vi "Autonomous.vi"   [LabVIEW 2016]
doc: "This VI starts when autonomous period begins, and will automatically be terminated when it ends. You can carry out timed or sensor driven operations directly to I/O or to subsystems without needing to return to the caller."
uses:
  <vilib>/Rock Robotics/WPI/Utilities/WPI_GetSetVariantRefNum.vi
  <vilib>/Rock Robotics/Network Tables/NT Read String.vi
types:
  T1 = typedef "WPI_DriverStationPositionInfo.ctl" = enum16{"1", "2", "3"}
  T2 = typedef "WPI_JoystickDevRef.ctl" = cluster{"Device":T3}
  T3 = typedef "WPI_JoystickDeviceEnum.ctl" = enum16{"USB 0", "USB 1", "USB 2", "USB 3", "USB 4", "USB 5"}
  T4 = typedef "Command Status Info.ctl" = cluster{"Name":string, "Status":T5, "notifier out":T6}
  T5 = typedef "Completion Status.ctl" = enum16{"Successful", "Aborted", "Incomplete"}
  T6 = typedef "Completion Notifier.ctl" = refnum<notifier>
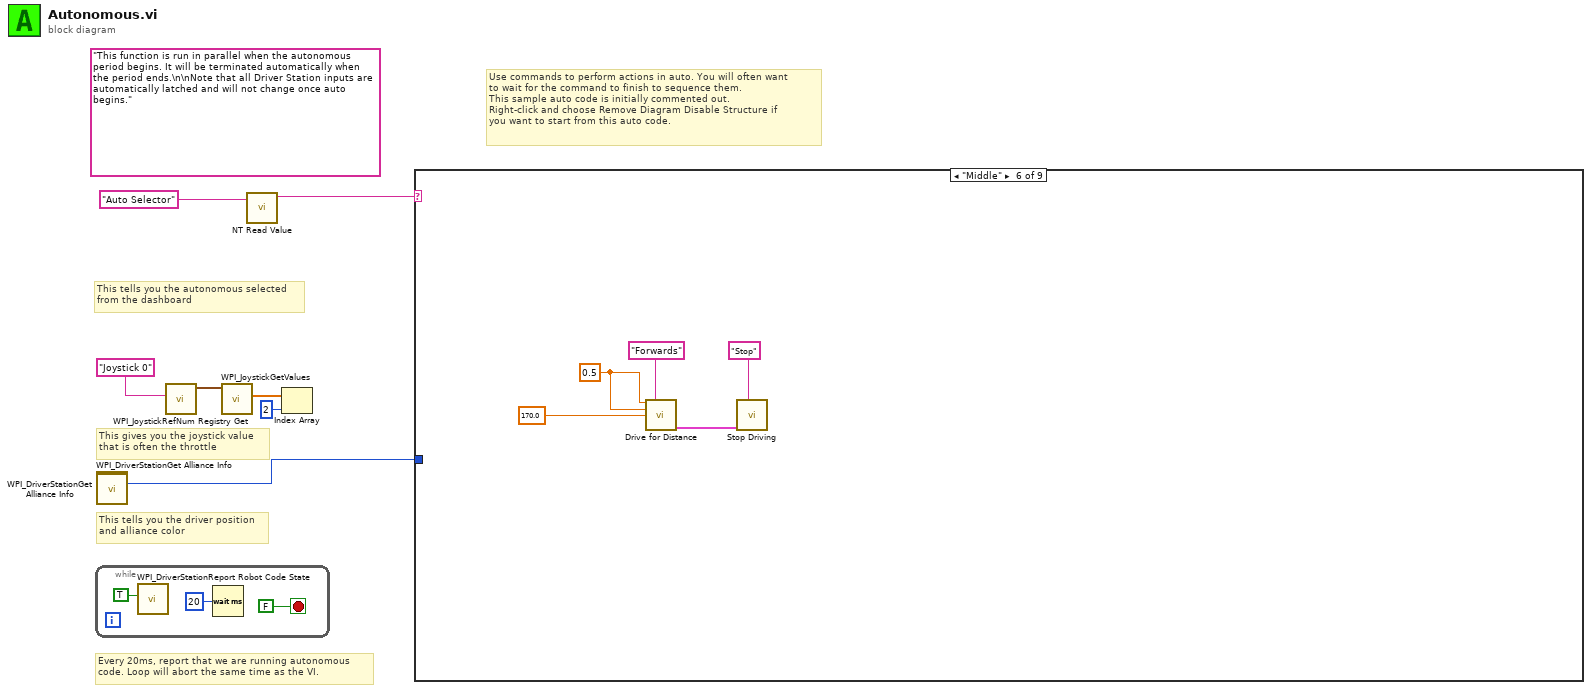
[diagram p0: block diagram]
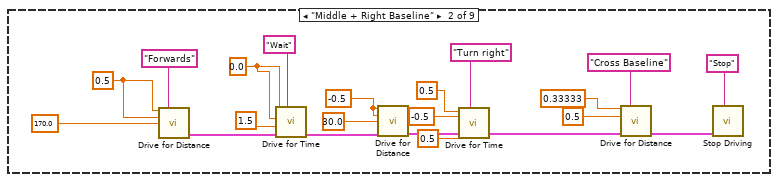
[diagram p3: hidden frame]
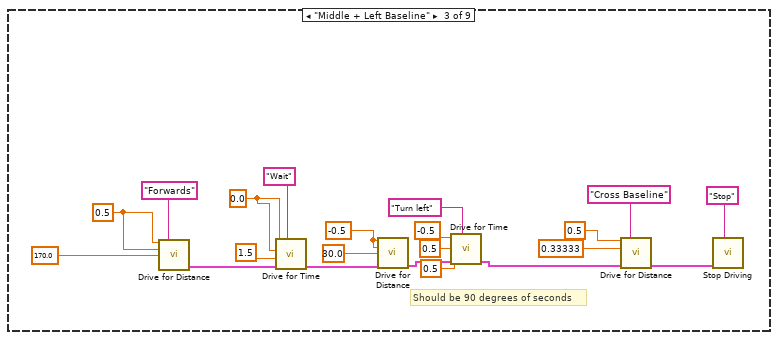
[diagram p4: hidden frame]
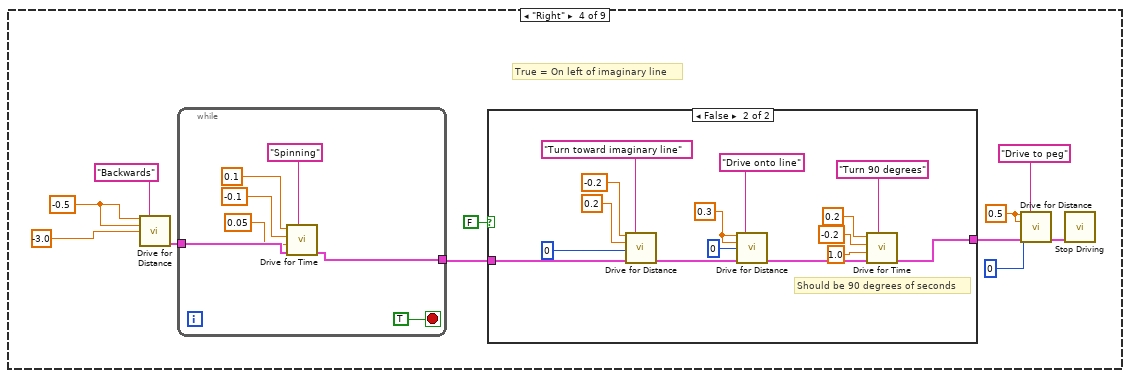
[diagram p5: hidden frame]
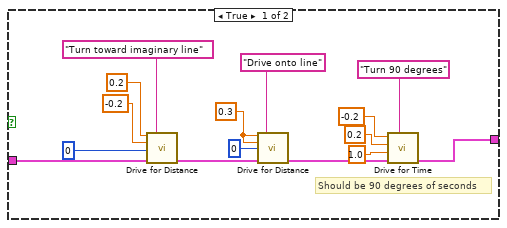
[diagram p6: hidden frame]
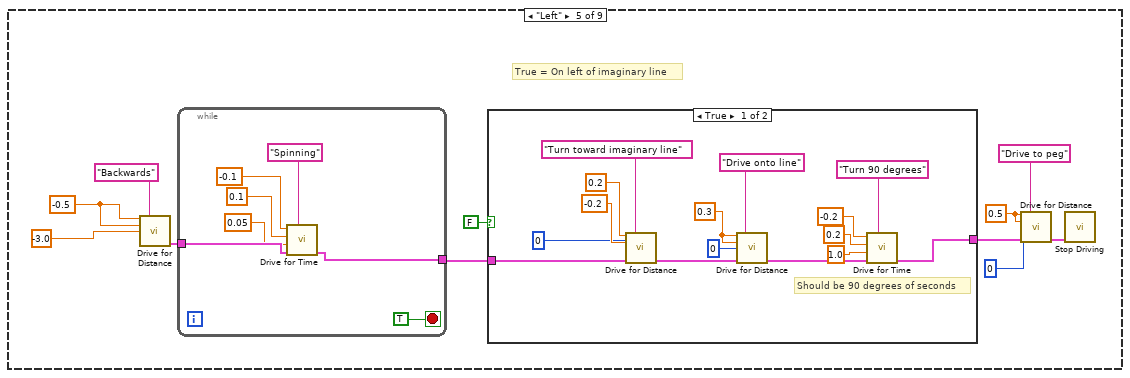
[diagram p7: hidden frame]
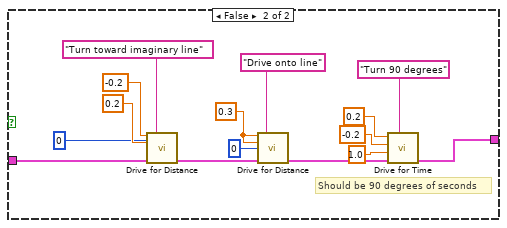
[diagram p8: hidden frame]
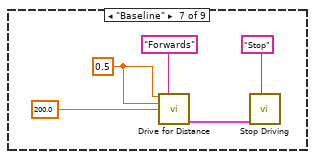
[diagram p9: hidden frame]
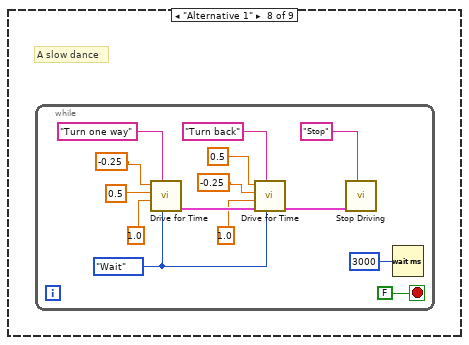
[diagram p10: hidden frame]
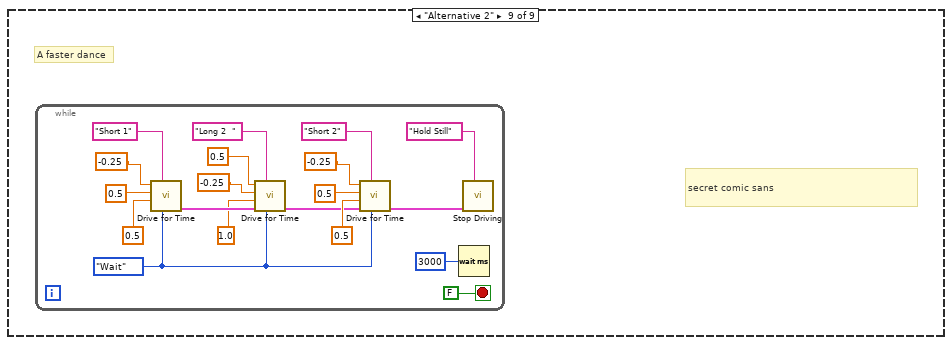
[diagram p11: hidden frame]
diagram:
  (unwired) "This function is run in parallel when the autonomous period begins. It will be terminated automatically when the period ends.\n\nNote that all Driver Station inputs are automatically latched and will not change once auto begins."
  # "This tells you the autonomous selected\nfrom the dashboard"
  # "Every 20ms, report that we are running autonomous\ncode. Loop will abort the same time as the VI."
  # "This gives you the joystick value\nthat is often the throttle"
  # "Use commands to perform actions in auto. You will often want\nto wait for the command to finish to sequence them.\nThis sample auto code is initially commented out. \nRight-click and choose Remove Diagram Disable Structure if\nyou want to start from this auto code."
  # "This tells you the driver position\nand alliance color"
  n1 = while {
    stop <- FALSE stop-if-true
    n2 = call <vilib>:"WPI_DriverStationReport Robot Code State.vi"("Autonomous"=TRUE) -> ()  [unwired: 10 in, 1 out]
    n3 = Wait (ms)(milliseconds to wait=u32 20) -> ()  [unwired: 1 out]
  }
  n4 = call <vilib>:"WPI_DriverStationGet Alliance Info.vi"() -> ("Position"=w1:T1)  [unwired: 11 out]
  n5 = call <vilib>:"WPI_DriverStationGet Alliance Info.vi"() -> ()  [unwired: 12 out]
  n6 = call <vilib>:"WPI_JoystickRefNum Registry Get.vi"("refnum name"="Joystick 0") -> ("JoystickDevRef"=w6:T2)  [unwired: 1 in, 9 out]
  n7 = call <vilib>:"WPI_JoystickGetValues.vi"("JoystickDevRef"=w6) -> ("Axes"=w5:dbl[])  [unwired: 6 in, 4 out]
  n8 = call-poly <vilib>:"NT Read Value.vi"("Name"="Auto Selector") -> ("String"=w2:string)  [unwired: 9 in, 1 out]
  n9 = Index Array(array=w5, index=2) -> ()  [unwired: 1 out]
  n10 = case shown="\"Middle\"" w2 {
    tunnel: w1 -> [_ _ _ _ _ _ _ _ _]
    frame Default {
      # "You can put your main auto here, or you can right-click on the case and make any\nother frame be the default case."
      # "This is the frame that will execute if no selection is made, or if it is not recognized"
    }
    frame "Middle + Right Baseline" {
      w22 = -0.5 ("Left Setpoint")
      w25 = 0.0 ("Left Speed")
      w30 = 0.5
      n11 = call "Drive for Distance.vi"("Left Setpoint"=w30, "Description"="Forwards", "Right Setpoint"=w30, "Distance"=170.0) -> ("Command Info Out"=w27:T4)  [unwired: 11 in]
      n12 = call "Drive for Time.vi"("Description"="Wait", "Command Info In"=w27, "Seconds"=1.5, "Right Speed"=w25, "Left Speed"=w25) -> ("Command Info Out"=w21:T4)  [unwired: 5 in, 1 out]
      n13 = call "Drive for Distance.vi"("Left Setpoint"=w22, "Right Setpoint"=w22, "Distance"=30.0, "Command Info In"=w21) -> ("Command Info Out"=w16:T4)  [unwired: 11 in]
      n14 = call "Drive for Time.vi"("Description"="Turn right", "Command Info In"=w16, "Seconds"=0.5, "Right Speed"=-0.5 ("Angle"), "Left Speed"=0.5 ("Setpoint")) -> ("Command Info Out"=w12:T4)  [unwired: 5 in, 1 out]
      n15 = call "Drive for Distance.vi"("Left Setpoint"=0.33333, "Description"="Cross Baseline", "Right Setpoint"=0.5, "Command Info In"=w12) -> ("Command Info Out"=w17:T4)  [unwired: 11 in]
      n16 = call "Stop Driving.vi"("Description"="Stop", "Command Info In"=w17) -> ()  [unwired: 9 in, 1 out]
    }
    frame "Middle + Left Baseline" {
      w43 = -0.5 ("Left Setpoint")
      w46 = 0.0 ("Left Speed")
      w51 = 0.5
      # "Should be 90 degrees of seconds"
      n17 = call "Drive for Distance.vi"("Left Setpoint"=w51, "Description"="Forwards", "Right Setpoint"=w51, "Distance"=170.0) -> ("Command Info Out"=w48:T4)  [unwired: 11 in]
      n18 = call "Drive for Time.vi"("Description"="Wait", "Command Info In"=w48, "Seconds"=1.5, "Right Speed"=w46, "Left Speed"=w46) -> ("Command Info Out"=w42:T4)  [unwired: 5 in, 1 out]
      n19 = call "Drive for Distance.vi"("Left Setpoint"=w43, "Right Setpoint"=w43, "Distance"=30.0, "Command Info In"=w42) -> ("Command Info Out"=w37:T4)  [unwired: 11 in]
      n20 = call "Drive for Time.vi"("Description"="Turn left", "Command Info In"=w37, "Seconds"=0.5, "Right Speed"=0.5 ("Angle"), "Left Speed"=-0.5 ("Setpoint")) -> ("Command Info Out"=w36:T4)  [unwired: 5 in, 1 out]
      n21 = call "Drive for Distance.vi"("Left Setpoint"=0.5, "Description"="Cross Baseline", "Right Setpoint"=0.33333, "Command Info In"=w36) -> ("Command Info Out"=w38:T4)  [unwired: 11 in]
      n22 = call "Stop Driving.vi"("Description"="Stop", "Command Info In"=w38) -> ()  [unwired: 9 in, 1 out]
    }
    frame "Right" {
      w56 = 0.5 ("Left Setpoint")
      w62 = -0.5 ("Left Setpoint")
      # "True = On left of imaginary line"
      n23 = call "Drive for Distance.vi"("Left Setpoint"=w62, "Description"="Backwards", "Right Setpoint"=w62, "Distance"=-3.0) -> ("Command Info Out"=w60:T4)  [unwired: 11 in]
      n24 = while {
        tunnel: w60 -> [w100]
        tunnel: [w95] -> w59
        stop <- TRUE stop-if-true
        n25 = call "Drive for Time.vi"("Description"="Spinning", "Command Info In"=w100, "Seconds"=0.05, "Right Speed"=-0.1 ("Right Setpoint"), "Left Speed"=0.1 ("Left Setpoint")) -> ("Command Info Out"=w95:T4)  [unwired: 5 in, 1 out]
      }
      n26 = case shown="False" FALSE {
        tunnel: w59 -> [w78 w93]
        tunnel: [w64 w79] -> w57
        frame True {
          w70 = 0.3 ("Left Setpoint")
          # "Should be 90 degrees of seconds"
          n27 = call "Drive for Distance.vi"("Left Setpoint"=0.2, "Description"="Turn toward imaginary line", "Right Setpoint"=-0.2, "Distance"=0 ("temp (from vision)"), "Command Info In"=w78) -> ("Command Info Out"=w66:T4)  [unwired: 10 in]
          n28 = call "Drive for Distance.vi"("Left Setpoint"=w70, "Description"="Drive onto line", "Right Setpoint"=w70, "Distance"=0, "Command Info In"=w66) -> ("Command Info Out"=w72:T4)  [unwired: 10 in]
          n29 = call "Drive for Time.vi"("Description"="Turn 90 degrees", "Command Info In"=w72, "Seconds"=1.0, "Right Speed"=0.2 ("Right Setpoint"), "Left Speed"=-0.2 ("Left Setpoint")) -> ("Command Info Out"=w64:T4)  [unwired: 5 in, 1 out]
        }
        frame False {
          w85 = 0.3 ("Left Setpoint")
          # "Should be 90 degrees of seconds"
          n30 = call "Drive for Distance.vi"("Left Setpoint"=-0.2, "Description"="Turn toward imaginary line", "Right Setpoint"=0.2, "Distance"=0 ("temp (from vision)"), "Command Info In"=w93) -> ("Command Info Out"=w81:T4)  [unwired: 10 in]
          n31 = call "Drive for Distance.vi"("Left Setpoint"=w85, "Description"="Drive onto line", "Right Setpoint"=w85, "Distance"=0, "Command Info In"=w81) -> ("Command Info Out"=w87:T4)  [unwired: 10 in]
          n32 = call "Drive for Time.vi"("Description"="Turn 90 degrees", "Command Info In"=w87, "Seconds"=1.0, "Right Speed"=-0.2 ("Right Setpoint"), "Left Speed"=0.2 ("Left Setpoint")) -> ("Command Info Out"=w79:T4)  [unwired: 5 in, 1 out]
        }
      }
      n33 = call "Drive for Distance.vi"("Left Setpoint"=w56, "Description"="Drive to peg", "Right Setpoint"=w56, "Distance"=0, "Command Info In"=w57) -> ("Command Info Out"=w54:T4)  [unwired: 10 in]
      n34 = call "Stop Driving.vi"("Command Info In"=w54) -> ()  [unwired: 10 in, 1 out]
    }
    frame "Left" {
      w104 = 0.5 ("Left Setpoint")
      w110 = -0.5 ("Left Setpoint")
      # "True = On left of imaginary line"
      n35 = call "Drive for Distance.vi"("Left Setpoint"=w110, "Description"="Backwards", "Right Setpoint"=w110, "Distance"=-3.0) -> ("Command Info Out"=w108:T4)  [unwired: 11 in]
      n36 = while {
        tunnel: w108 -> [w148]
        tunnel: [w143] -> w107
        stop <- TRUE stop-if-true
        n37 = call "Drive for Time.vi"("Description"="Spinning", "Command Info In"=w148, "Seconds"=0.05, "Right Speed"=0.1 ("Right Setpoint"), "Left Speed"=-0.1 ("Left Setpoint")) -> ("Command Info Out"=w143:T4)  [unwired: 5 in, 1 out]
      }
      n38 = case shown="True" FALSE {
        tunnel: w107 -> [w126 w141]
        tunnel: [w112 w127] -> w105
        frame True {
          w118 = 0.3 ("Left Setpoint")
          # "Should be 90 degrees of seconds"
          n39 = call "Drive for Distance.vi"("Left Setpoint"=0.2, "Description"="Turn toward imaginary line", "Right Setpoint"=-0.2, "Distance"=0 ("temp (from vision)"), "Command Info In"=w126) -> ("Command Info Out"=w114:T4)  [unwired: 10 in]
          n40 = call "Drive for Distance.vi"("Left Setpoint"=w118, "Description"="Drive onto line", "Right Setpoint"=w118, "Distance"=0, "Command Info In"=w114) -> ("Command Info Out"=w120:T4)  [unwired: 10 in]
          n41 = call "Drive for Time.vi"("Description"="Turn 90 degrees", "Command Info In"=w120, "Seconds"=1.0, "Right Speed"=0.2 ("Right Setpoint"), "Left Speed"=-0.2 ("Left Setpoint")) -> ("Command Info Out"=w112:T4)  [unwired: 5 in, 1 out]
        }
        frame False {
          w133 = 0.3 ("Left Setpoint")
          # "Should be 90 degrees of seconds"
          n42 = call "Drive for Distance.vi"("Left Setpoint"=-0.2, "Description"="Turn toward imaginary line", "Right Setpoint"=0.2, "Distance"=0 ("temp (from vision)"), "Command Info In"=w141) -> ("Command Info Out"=w129:T4)  [unwired: 10 in]
          n43 = call "Drive for Distance.vi"("Left Setpoint"=w133, "Description"="Drive onto line", "Right Setpoint"=w133, "Distance"=0, "Command Info In"=w129) -> ("Command Info Out"=w135:T4)  [unwired: 10 in]
          n44 = call "Drive for Time.vi"("Description"="Turn 90 degrees", "Command Info In"=w135, "Seconds"=1.0, "Right Speed"=-0.2 ("Right Setpoint"), "Left Speed"=0.2 ("Left Setpoint")) -> ("Command Info Out"=w127:T4)  [unwired: 5 in, 1 out]
        }
      }
      n45 = call "Drive for Distance.vi"("Left Setpoint"=w104, "Description"="Drive to peg", "Right Setpoint"=w104, "Distance"=0, "Command Info In"=w105) -> ("Command Info Out"=w102:T4)  [unwired: 10 in]
      n46 = call "Stop Driving.vi"("Command Info In"=w102) -> ()  [unwired: 10 in, 1 out]
    }
    frame "Middle" {
      w152 = 0.5
      n47 = call "Drive for Distance.vi"("Left Setpoint"=w152, "Description"="Forwards", "Right Setpoint"=w152, "Distance"=170.0) -> ("Command Info Out"=w149:T4)  [unwired: 11 in]
      n48 = call "Stop Driving.vi"("Description"="Stop", "Command Info In"=w149) -> ()  [unwired: 9 in, 1 out]
    }
    frame "Baseline" {
      w157 = 0.5
      n49 = call "Drive for Distance.vi"("Left Setpoint"=w157, "Description"="Forwards", "Right Setpoint"=w157, "Distance"=200.0) -> ("Command Info Out"=w154:T4)  [unwired: 11 in]
      n50 = call "Stop Driving.vi"("Description"="Stop", "Command Info In"=w154) -> ()  [unwired: 9 in, 1 out]
    }
    frame "Alternative 1" {
      # "A slow dance"
      n51 = while {
        stop <- FALSE stop-if-true
        w163 = enum16{"Start", "Wait"}."Wait" ("Synchronication")
        n52 = call "Drive for Time.vi"("Synchronization"=w163, "Description"="Turn one way", "Seconds"=1.0 ("Delay (s)"), "Right Speed"=0.5 ("X axis value"), "Left Speed"=-0.25 ("X axis value")) -> ("Command Info Out"=w172:T4)  [unwired: 5 in, 1 out]
        n53 = call "Drive for Time.vi"("Synchronization"=w163, "Description"="Turn back", "Command Info In"=w172, "Seconds"=1.0 ("Delay (s)"), "Right Speed"=-0.25 ("X axis value"), "Left Speed"=0.5 ("X axis value")) -> ("Command Info Out"=w162:T4)  [unwired: 4 in, 1 out]
        n54 = call "Stop Driving.vi"("Description"="Stop", "Command Info In"=w162) -> ()  [unwired: 9 in, 1 out]
        n55 = Wait (ms)(milliseconds to wait=u32 3000 ("millisecond timer value")) -> ()  [unwired: 1 out]
      }
    }
    frame "Alternative 2" {
      # "secret comic sans"
      # "A faster dance"
      n56 = while {
        stop <- FALSE stop-if-true
        w173 = enum16{"Start", "Wait"}."Wait" ("Synchronication")
        n57 = call "Drive for Time.vi"("Synchronization"=w173, "Description"="Short 1", "Seconds"=0.5 ("Delay (s)"), "Right Speed"=0.5 ("X axis value"), "Left Speed"=-0.25 ("X axis value")) -> ("Command Info Out"=w191:T4)  [unwired: 5 in, 1 out]
        n58 = call "Drive for Time.vi"("Synchronization"=w173, "Description"="Long 2  ", "Command Info In"=w191, "Seconds"=1.0 ("Delay (s)"), "Right Speed"=-0.25 ("X axis value"), "Left Speed"=0.5 ("X axis value")) -> ("Command Info Out"=w175:T4)  [unwired: 4 in, 1 out]
        n59 = call "Drive for Time.vi"("Synchronization"=w173, "Description"="Short 2", "Command Info In"=w175, "Seconds"=0.5 ("Delay (s)"), "Right Speed"=0.5 ("X axis value"), "Left Speed"=-0.25 ("X axis value")) -> ("Command Info Out"=w174:T4)  [unwired: 4 in, 1 out]
        n60 = Wait (ms)(milliseconds to wait=u32 3000 ("millisecond timer value")) -> ()  [unwired: 1 out]
        n61 = call "Stop Driving.vi"("Description"="Hold Still", "Command Info In"=w174) -> ()  [unwired: 9 in, 1 out]
      }
    }
  }
